vi "Initialize Logger Queue.vi"(8 "error in (no error)":errorcluster, 11 "Test Number and Bin Generator in":refnum<class "Test Number and Bin Generator.lvclass">=refnum) -> (0 "error out":errorcluster, 3 "Test Number and Bin Generator out":refnum<class "Test Number and Bin Generator.lvclass">)   [LabVIEW 2018, in "Test Number and Bin Generator.lvlib" / "Test Number and Bin Generator.lvclass"]
uses:
  Test Number and Bin Generator.lvclass
  Test Number and Bin Generator.lvclass/Test Number and Bin Generator.ctl
  Typedefs/Evaluation QMH.ctl
  Plugins/TestStand API Tools (TSAT).lvlibp/Evaluation Actions/Includes/Controls/TSAT Eval SI Unit Scaling.ctl
  Plugins/TestStand API Tools (TSAT).lvlibp/Evaluation Actions/Includes/Controls/TSAT Evaluation Type.ctl
  Plugins/TestStand API Tools (TSAT).lvlibp/Evaluation Actions/TSAT Evaluation Actions.lvlib
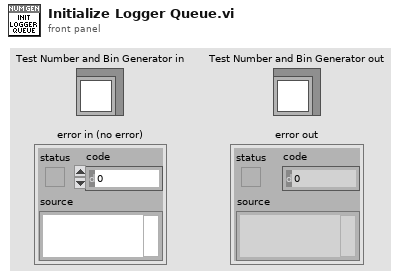
[diagram p1: front panel]
types:
  T1 = typedef "Test Number and Bin Generator.lvlib/Test Number and Bin Generator.lvclass/Evaluation QMH.ctl" = cluster{"Command":string, "Evaluations":cluster{"Test Name":string, "Pin":string, "Units":string, "SI Scaling":T2, "Test Number":i32, "Published Data Id":string, "Low Limit":dbl, "High Limit":dbl, "Export Data Location":string, "Software Bin":i64, "Evaluation Type":T3, "Test Data Source":string}[]}
  T2 = typedef "TestStand API Tools (TSAT).lvlibp/TSAT Evaluation Actions.lvlib/TSAT Eval SI Unit Scaling.ctl" = i16
  T3 = typedef "TestStand API Tools (TSAT).lvlibp/TSAT Evaluation Actions.lvlib/TSAT Evaluation Type.ctl" = enum16{"Numeric Limit", "Pass/Fail", "None"}
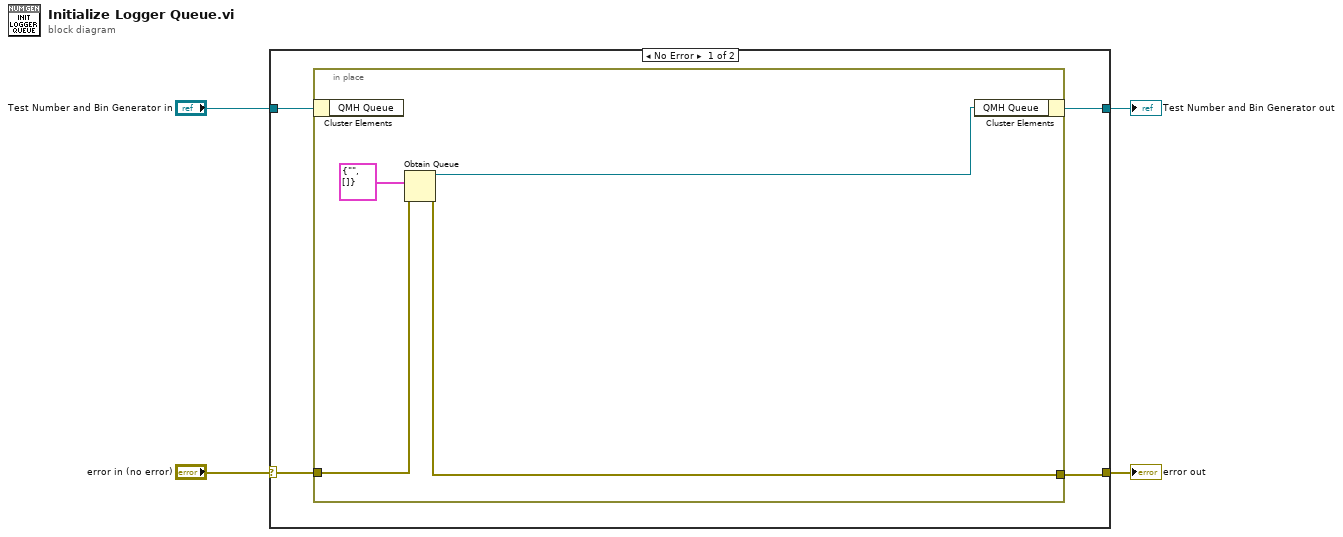
[diagram p0: block diagram]
diagram:
  n1 = case shown="No Error" "error in (no error)" {
    selector: "error in (no error)" -> [w6 w14]
    tunnel: [w5 w14] -> w3
    tunnel: [w7 w13] -> w1
    tunnel: "Test Number and Bin Generator in" -> [w8 w13]
    frame No Error {
      n2 = in-place {
        in-place-border: w6 -> [w11]
        in-place-border: [w10] -> w5
        n3 = in-place-cluster #1(w8) -> ()  [unwired: 1 out]
        n4 = Obtain Queue(element data type=T1 {"Command"="", "Evaluations"=[]} ("Evaluation QMH"), error in (no error)=w11) -> (queue out=w9:refnum<queue>, error out=w10:errorcluster)  [unwired: 3 in, 1 out]
        n5 = in-place-cluster #1("QMH Queue"=w9) -> (w7:refnum<class "Test Number and Bin Generator.lvclass">)
      }
    }
    frame Error {
    }
  }
  "error out" <- w3
  "Test Number and Bin Generator out" <- w1
